vi "ServerWrite.vi"(8 "error in":errorcluster, 10 "String \nInput":string, 11 "connection ID":refnum<k5>) -> (0 "error out":errorcluster)   [LabVIEW 2023]
panel:
  # "Output"
  # "Input"
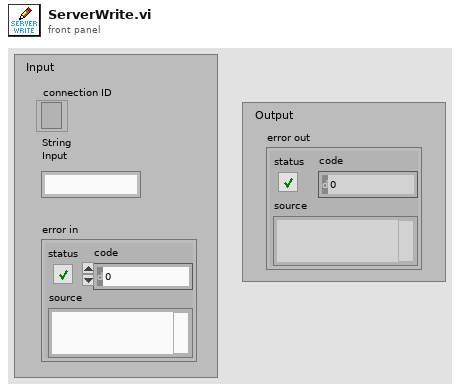
[diagram p1: front panel]
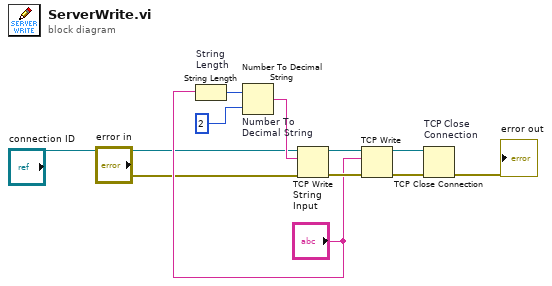
[diagram p0: block diagram]
diagram:
  n1 = String Length "String \nLength"(string="String \nInput") -> (length=w6:i32)
  n2 = Number To Decimal String "Number To \nDecimal String"(number=w6, width (-)=i16 2) -> (decimal integer string=w8:string)
  n3 = TCP Write(connection ID="connection ID", data in=w8, error in (no error)="error in") -> (connection ID out=w5:refnum<k5>, error out=w10:errorcluster)  [unwired: 1 in, 1 out]
  n4 = TCP Write(connection ID=w5, data in="String \nInput", error in (no error)=w10) -> (connection ID out=w11:refnum<k5>, error out=w9:errorcluster)  [unwired: 1 in, 1 out]
  n5 = TCP Close Connection "TCP Close \nConnection"(connection ID=w11, error in (no error)=w9) -> (error out=→"error out":errorcluster)  [unwired: 1 in, 1 out]
